vi "Get Server Connection Info.vi"(7 "Override Address":bool, 8 "error in":errorcluster, 11 "Default Address":string) -> (0 "error out":errorcluster, 3 "Server Connection":string)   [LabVIEW 2021, in "Python Orchestration.lvlib"]
uses:
  Python Orchestration.lvlib
  CIFConfigurationFile/CIF Configuration File.lvlib
  CIFCore/Common/CIFCoreCommon.lvlib
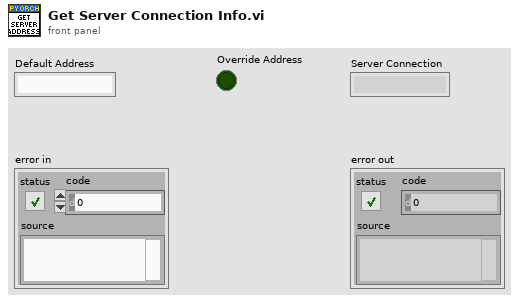
[diagram p1: front panel]
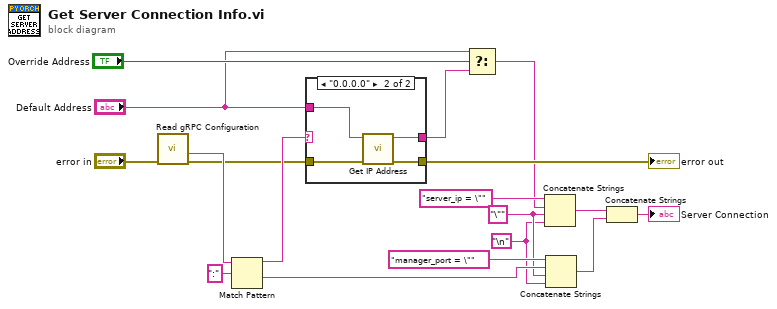
[diagram p0: block diagram]
diagram:
  w11 = "\n"
  w12 = "\"" ("string")
  n1 = call "Read gRPC Configuration.vi"("error in"="error in") -> ("error out"=w8:errorcluster, "Manager Server Address"=w18:string)  [unwired: 5 in, 4 out]
  n2 = Match Pattern(string=w18, regular expression=":") -> (before substring=w16:string, after substring=w13:string)  [unwired: 1 in, 2 out]
  n3 = case shown="\"0.0.0.0\"" w16 {
    selector: w16 -> [w20 _]
    tunnel: [w20 w24] -> w3
    tunnel: w8 -> [w19 w23]
    tunnel: [w19 w22] -> w7
    tunnel: "Default Address" -> [_ w21]
    frame "False", Default {
    }
    frame "0.0.0.0" {
      n4 = call "Get IP Address.vi"("error in (no error)"=w23, "Default Address"=w21) -> ("error out"=w22:errorcluster, "IPv4 Address"=w24:string)  [unwired: 8 in]
    }
  }
  "error out" <- w7
  n5 = Select(t="Default Address", s="Override Address", f=w3) -> (s? t:f=w1:string)
  n6 = Concatenate Strings("server_ip = \"" ("string"), w1, w12, w11) -> (w9:string)
  n7 = Concatenate Strings("manager_port = \"" ("string"), w13, w12, w11) -> (w10:string)
  n8 = Concatenate Strings(w9, w10) -> (→"Server Connection":string)
